vi "Match Cluster to Field.vi"(6 "path to png file":path=path "C:/Users/a0272913/Desktop/AppRawJSON/drawing.png", 10 "Wait on OK? (T)":bool=TRUE, 11 "JSONCluster":T1) -> (2 "Cancelled?":bool, 3 "Field":picture)   [LabVIEW 2015]
uses:
  Typedef/JSONCluster.ctl
panel:
  in  "Cancel Button":bool
  in  "OK Button":bool
  out "Match Number":i32
  out "Team Number":i32
  # "Team Number:"
  # "Match Number:"
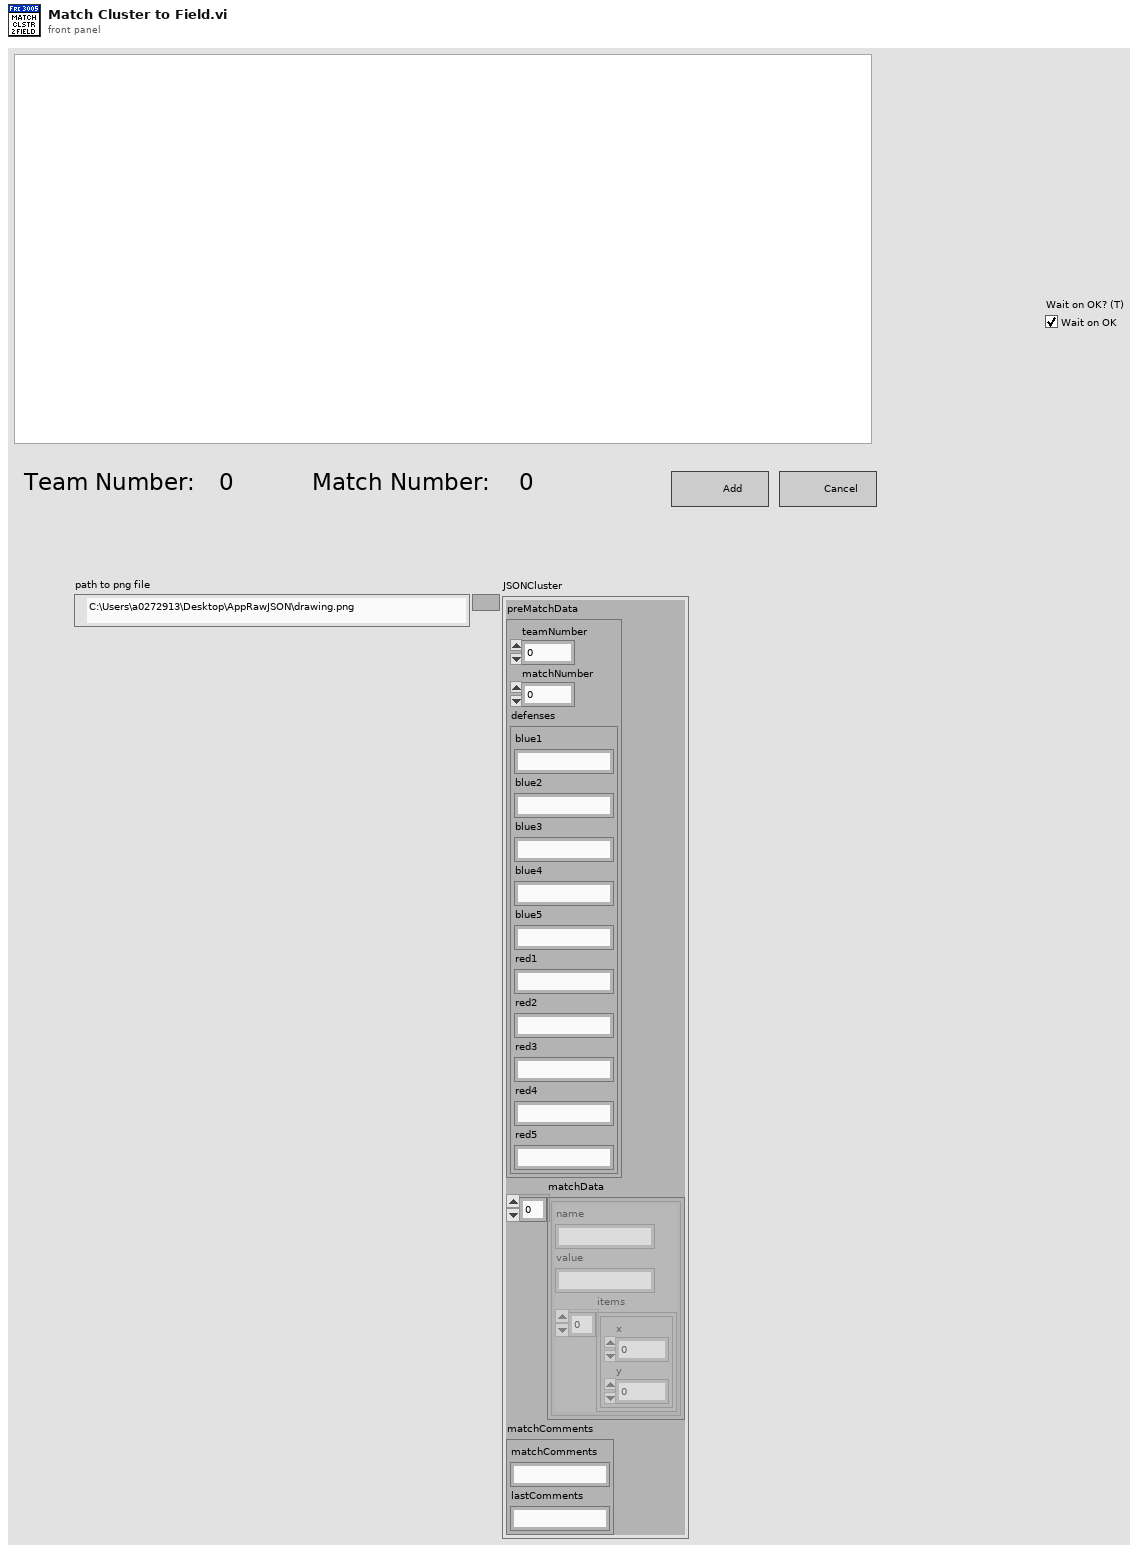
[diagram p1: front panel]
types:
  T1 = typedef "JSONCluster.ctl" = cluster{"preMatchData":cluster{"teamNumber":i32, "matchNumber":i32, "defenses":cluster{"blue1":string, "blue2":string, "blue3":string, "blue4":string, "blue5":string, "red1":string, "red2":string, "red3":string, "red4":string, "red5":string}}, "matchData":cluster{"name":string, "value":string, "items":cluster{"x":i32, "y":i32}[]}[], "matchComments":cluster{"matchComments":string, "lastComments":string}}
  T2 = typedef "LVBoundsTypeDef.ctl" = cluster{"Width":u32, "Height":u32}
  T3 = typedef "imagedata.ctl" = cluster{"image type":i32, "image depth":i32, "image":u8[], "mask":u8[], "colors":u32[], "Rectangle":cluster{"left":i16, "top":i16, "right":i16, "bottom":i16}}
  T4 = cluster{"teamNumber":i32, "matchNumber":i32, "defenses":cluster{"blue1":string, "blue2":string, "blue3":string, "blue4":string, "blue5":string, "red1":string, "red2":string, "red3":string, "red4":string, "red5":string}}
  T5 = cluster{"name":string, "value":string, "items":cluster{"x":i32, "y":i32}[]}[]
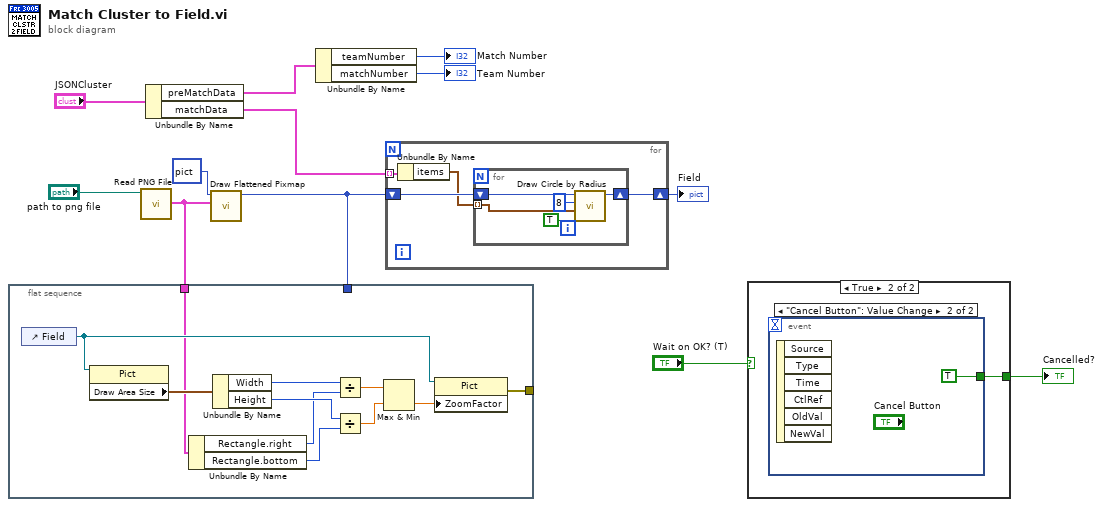
[diagram p0: block diagram]
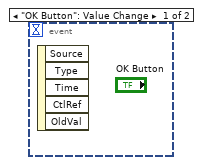
[diagram p3: hidden frame]
diagram:
  n1 = flat-sequence {
    tunnel: w11 -> [w14]
    tunnel: [w13] -> _
    tunnel: w6 -> [_]
    frame #0 {
      n2 = control-ref of="Field"() -> (w15:refnum<vi>)
      n3 = property class="Pict"(reference=w15) -> ("Draw Area Size"=w20:T2)  [unwired: 1 in, 2 out]
      n4 = Unbundle By Name(w14) -> ("Rectangle.right"=w17:i16, "Rectangle.bottom"=w16:i16)
      n5 = Unbundle By Name(w20) -> ("Width"=w19:u32, "Height"=w18:u32)
      n6 = Divide(x=w19, y=w17) -> (x/y=w21:dbl)
      n7 = Divide(x=w18, y=w16) -> (x/y=w22:dbl)
      n8 = Max & Min(x=w21, y=w22) -> (min(x,y)=w23:dbl)  [unwired: 1 out]
      n9 = property class="Pict"(reference=w15, "ZoomFactor"=w23) -> (error out=w13:errorcluster)  [unwired: 1 in, 1 out]
    }
  }
  n10 = call <vilib>:"Read PNG File.vi"("path to PNG file"="path to png file") -> ("image data"=w11:T3)  [unwired: 8 in, 2 out]
  n11 = Unbundle By Name("JSONCluster") -> ("preMatchData"=w7:T4, "matchData"=w9:T5)
  n12 = call <vilib>:"Draw Flattened Pixmap.vi"("image data"=w11, "picture"=picture data[5B]) -> ("new picture"=w6:picture)  [unwired: 7 in]
  n13 = Unbundle By Name(w7) -> ("teamNumber"=→"Match Number":i32, "matchNumber"=→"Team Number":i32)
  n14 = for {
    shift-right: [w26] -> w10
    shift-left: w6 -> [w27]
    tunnel: w9 -> [w25] mode=indexing
    n15 = Unbundle By Name(w25) -> ("items"=w24:cluster{"x":i32, "y":i32}[])
    n16 = for {
      shift-right: [w31] -> w26
      shift-left: w27 -> [w32]
      tunnel: w24 -> [w30] mode=indexing
      n17 = call <vilib>:"Draw Circle by Radius.vi"("fill?(F)"=TRUE, "pixel center"=w30, "radius"=i16 8, "picture"=w32) -> ("new picture"=w31:picture)  [unwired: 7 in]
    }
  }
  "Field" <- w10
  n18 = case shown="True" "Wait on OK? (T)" {
    tunnel: [_ w33] -> w1
    frame False {
    }
    frame True {
      n19 = event shown="[1] \"Cancel Button\": Value Change" {
        selector: _ -> [_ _]
        dyn-events: _ -> [_ _]
        timeout: _ -> [_ _]
        tunnel: [_ TRUE] -> w33
        event "OK Button": Value Change {
          n20 = event-data() -> ()  [unwired: 1 in, 5 out]
        }
        event "Cancel Button": Value Change {
          n21 = event-data() -> ()  [unwired: 1 in, 6 out]
        }
      }
    }
  }
  "Cancelled?" <- w1
